vi "OutputGripper.vi"   [LabVIEW 2020]
uses:
  GlobalGripper.vi
  GRNF_GenericSolenoid.vi
  TAI_Solenoid.vi
  <vilib>/Rock Robotics/WPI/Solenoid/Deprecated/WPI_SolenoidSetBool.vi
types:
  T1 = typedef "WPI_SolenoidDevRef.ctl" = cluster{"DevStatus":errorcluster, "Pneumatics Control Module":u8, "Forward Solenoid Channel":T2, "Reverse Solenoid Channel":T2}
  T2 = typedef "WPI_SolenoidChannel.ctl" = enum8{"Solenoid 0", "Solenoid 1", "Solenoid 2", "Solenoid 3", "Solenoid 4", "Solenoid 5", "Solenoid 6", "Solenoid 7", "Solenoid 8", "Solenoid 9", "Solenoid 10", "Solenoid 11", "Solenoid 12", "Solenoid 13", "Solenoid 14", "Solenoid 15", "Invalid"}
  T3 = enum16{"No Changed Output", "New Normal Output", "New Testing Output"}
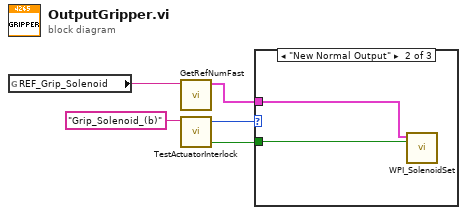
[diagram p0: block diagram]
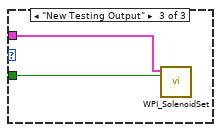
[diagram p3: hidden frame]
diagram:
  n1 = global read "GlobalGripper.vi" "REF_Grip_Solenoid"() -> (w1:string)
  n2 = call-poly "GetRefNumFast.vi"("RefNum Name"=w1) -> ("Device Reference"=w2:T1)  [unwired: 5 in, 1 out]
  n3 = call-poly "TestActuatorInterlock.vi"("Actuator Name"="Grip_Solenoid_(b)" ("Actuator_Name")) -> ("Interlocked Output"=w3:bool, "Output Mode"=w4:T3)  [unwired: 4 in]
  n4 = case shown="\"New Normal Output\"" w4 {
    tunnel: w3 -> [_ w6 w8]
    tunnel: w2 -> [_ w7 w9]
    frame "No Changed Output", Default {
    }
    frame "New Normal Output" {
      n5 = call-poly <vilib>:"WPI_SolenoidSet.vi"("Value"=w6, "SolenoidDevRef"=w7) -> ()  [unwired: 8 in, 2 out]
    }
    frame "New Testing Output" {
      n6 = call-poly <vilib>:"WPI_SolenoidSet.vi"("Value"=w8, "SolenoidDevRef"=w9) -> ()  [unwired: 8 in, 2 out]
    }
  }
